vi "Simulated Filter Signal.vi"() -> ()   [LabVIEW 2015]
panel:
  in  "stop":bool
  in  "Slide 3":dbl(slide) scale=0.0..16000.0
  in  "Slide 2":dbl(slide) scale=0.0..3000.0
  in  "Slide":dbl(slide) scale=0.0..1200.0
  out "Waveform Graph 3":dynamicdata(graph)
  out "Waveform Graph 2":dynamicdata(graph)
  out "Waveform Graph":dynamicdata(graph)
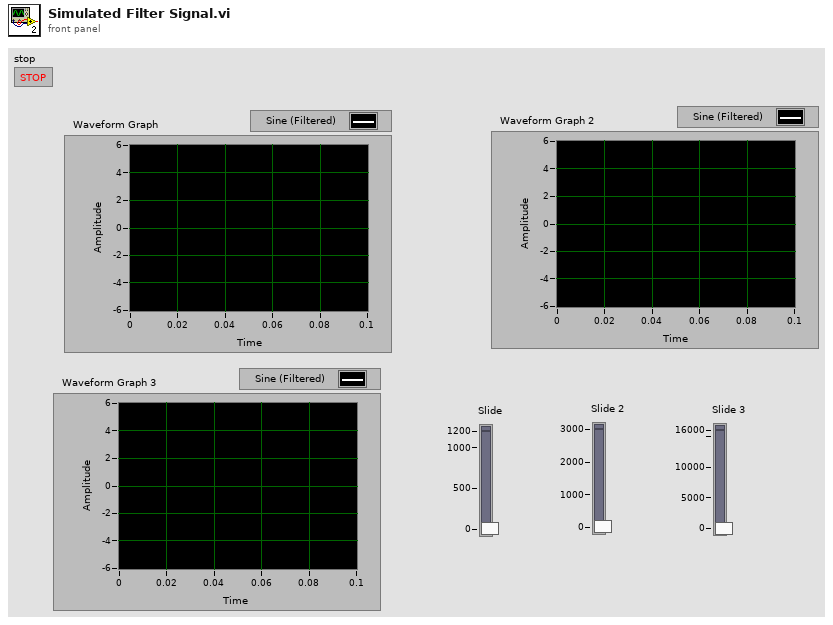
[diagram p1: front panel]
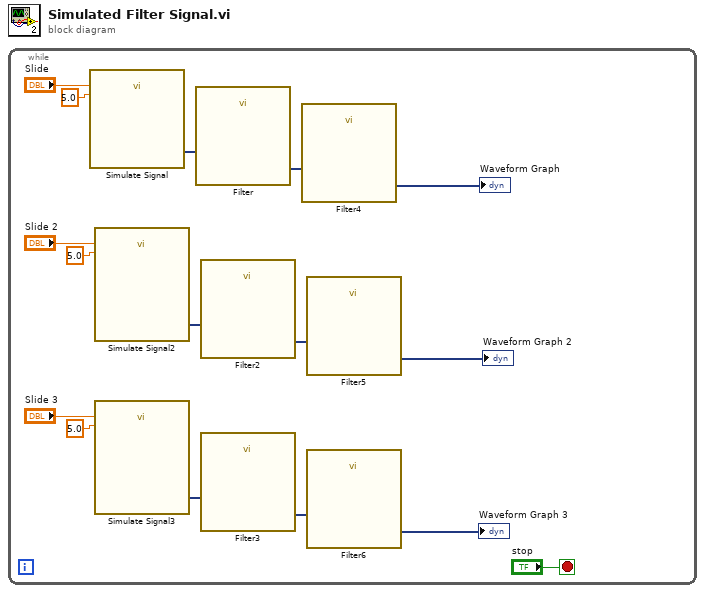
[diagram p0: block diagram]
diagram:
  n1 = while {
    stop <- "stop" stop-if-true
    n2 = call "Simulate Signal"("Frequency"="Slide", "Amplitude"=5.0) -> ("Sine"=w13:dynamicdata)  [unwired: 12 in, 1 out]
    n3 = call "Simulate Signal2"("Frequency"="Slide 2", "Amplitude"=5.0) -> ("Sine"=w12:dynamicdata)  [unwired: 12 in, 1 out]
    n4 = call "Simulate Signal3"("Frequency"="Slide 3", "Amplitude"=5.0) -> ("Sine"=w11:dynamicdata)  [unwired: 12 in, 1 out]
    n5 = call "Filter"("Signal"=w13) -> ("Filtered Signal"=w10:dynamicdata)  [unwired: 9 in, 1 out]
    n6 = call "Filter2"("Signal"=w12) -> ("Filtered Signal"=w9:dynamicdata)  [unwired: 9 in, 1 out]
    n7 = call "Filter3"("Signal"=w11) -> ("Filtered Signal"=w8:dynamicdata)  [unwired: 9 in, 1 out]
    n8 = call "Filter4"("Signal"=w10) -> ("Filtered Signal"=→"Waveform Graph":dynamicdata)  [unwired: 9 in, 1 out]
    n9 = call "Filter5"("Signal"=w9) -> ("Filtered Signal"=→"Waveform Graph 2":dynamicdata)  [unwired: 9 in, 1 out]
    n10 = call "Filter6"("Signal"=w8) -> ("Filtered Signal"=→"Waveform Graph 3":dynamicdata)  [unwired: 9 in, 1 out]
  }
